vi "readConfig.vi"(8 "error in (no error)":errorcluster, 9 "config":string, 10 "deviceName":string, 11 "K2602FileReader in":refnum<class "K2602FileReader.lvclass">) -> (0 "error out":errorcluster, 3 "K2602FileReader out":refnum<class "K2602FileReader.lvclass">)   [LabVIEW 2011, in "Tools.lvlib" / "Filing.lvlib" / "K2602FileReader.lvclass"]
uses:
  K2602FileReader.lvclass
  Hal/Channels/VoltOutput/AnalogOutput.lvclass
  K2602FileReader.lvclass/K2602FileReader.ctl
  FileReader.lvclass
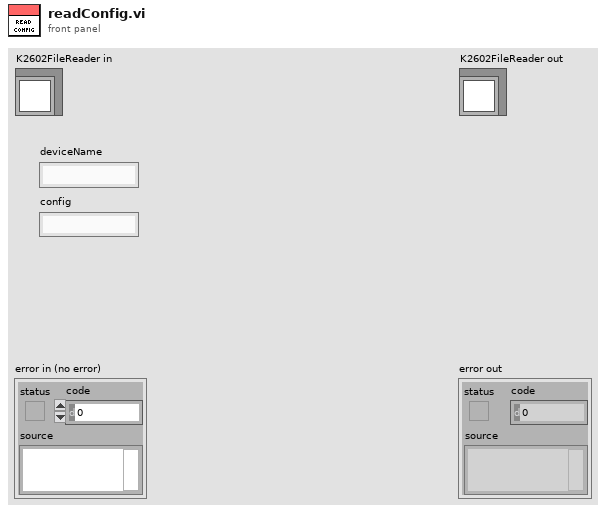
[diagram p1: front panel]
types:
  T1 = cluster{"Range":cluster{"current":dbl, "voltage":dbl}, "triggering_inUse":cluster{"start_trigger":string, "clock":string}, "Limits":cluster{"VoltageLimit":dbl, "CurrentLimit":dbl}}[]
  T2 = cluster{"clock":string, "start_trigger":string}[]
  T3 = cluster{"Range":cluster{"current":dbl, "voltage":dbl}, "triggering_inUse":cluster{"start_trigger":string, "clock":string}, "Limits":cluster{"VoltageLimit":dbl, "CurrentLimit":dbl}}
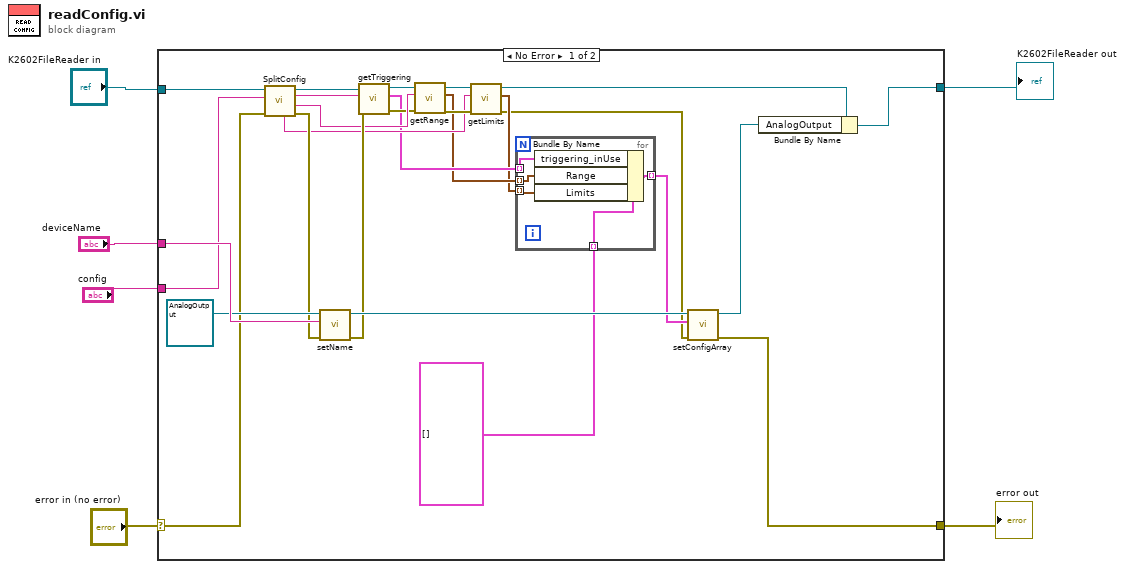
[diagram p0: block diagram]
diagram:
  n1 = case shown="No Error" "error in (no error)" {
    selector: "error in (no error)" -> [w29 w39]
    tunnel: [w30 w38] -> w5
    tunnel: [w7 w39] -> w4
    tunnel: "config" -> [w28 _]
    tunnel: "deviceName" -> [w32 _]
    tunnel: "K2602FileReader in" -> [w27 w38]
    frame No Error {
      n2 = call "SplitConfig.vi"("error in (no error)"=w29, "Config"=w28, "FileReader in"=w27) -> ("error out"=w24:errorcluster, "Range"=w20:string, "triggering"=w22:string, "FileReader out"=w25:refnum<class "K2602FileReader.lvclass">, "limits"=w15:string)  [unwired: 4 in]
      n3 = call "setName.vi"("error in (no error)"=w24, "name"=w32, "AnalogOutput.lvclass in"=refnum<class "AnalogOutput.lvclass"> refnum ("Hardware:Channels.lvlib:AnalogOutput.lvclass")) -> ("error out"=w23:errorcluster, "AnalogOutput.lvclass out"=w26:refnum<class "AnalogOutput.lvclass">)  [unwired: 7 in]
      n4 = call "getTriggering.vi"("error in (no error)"=w23, "triggering"=w22, "K2602FileReader in"=w25) -> ("error out"=w19:errorcluster, "triggering"=w14:T2, "K2602FileReader out"=w21:refnum<class "K2602FileReader.lvclass">)  [unwired: 6 in]
      n5 = call "getRange.vi"("error in (no error)"=w19, "config"=w20, "K2602FileReader in"=w21) -> ("error out"=w16:errorcluster, "range"=w13:cluster{"current":dbl, "voltage":dbl}[], "K2602FileReader out"=w18:refnum<class "K2602FileReader.lvclass">)  [unwired: 6 in]
      n6 = call "getLimits.vi"("error in (no error)"=w16, "config"=w15, "K2602FileReader in"=w18) -> ("error out"=w9:errorcluster, "limits"=w12:cluster{"current":dbl, "voltage":dbl}[], "K2602FileReader out"=w17:refnum<class "K2602FileReader.lvclass">)  [unwired: 6 in]
      n7 = for {
        tunnel: w14 -> [w34] mode=indexing
        tunnel: w13 -> [w33] mode=indexing
        tunnel: w12 -> [w37] mode=indexing
        tunnel: [w36] -> w10 mode=indexing
        tunnel: T1 [] ("ConfigArray") -> [w35] mode=indexing
        n8 = Bundle By Name(cluster=w35, "triggering_inUse"=w34, "Range"=w33, "Limits"=w37) -> (w36:T3)
      }
      n9 = call-dynamic "setConfigArray.vi"("error in (no error)"=w9, "ConfigArray"=w10, "AnalogOutput in"=w26) -> ("error out"=w7:errorcluster, "AnalogOutput out"=w8:refnum<class "AnalogOutput.lvclass">)  [unwired: 7 in]
      n10 = Bundle By Name(cluster=w17, "AnalogOutput"=w8) -> (w30:refnum<class "K2602FileReader.lvclass">)
    }
    frame Error {
    }
  }
  "error out" <- w4
  "K2602FileReader out" <- w5
